vi "GM_MyRIO(FPGA).vi"() -> ()   [LabVIEW 2017]
uses:
  <vilib>/rvi/Emulation/niFpgaGetClockAttributes.vi
  <vilib>/rvi/Emulation/niFpgaSctlEmulationGetInTimedLoop.vi
  <vilib>/rvi/Emulation/niFpgaEmulationReportErrorSimple.vi
  <vilib>/rvi/interface/RandomDataEmulation/niFpgaRandomDataHandleErrors.vi
  <vilib>/rvi/Memory/Memory_Emulation/nirvimemoryEmulation.vi
  <vilib>/rvi/Memory/Memory_Emulation/nirvimemoryFastEmulation.vi
  <vilib>/rvi/DataTransferAndStorage/Container/Common/niFpgaContainerGetUniqueNameForEmu.vi
  <vilib>/rvi/Memory/Memory_Emulation/niFpgaMemoryEmulationCacheClearOnFirstRun.vi
  <vilib>/rvi/Memory/Memory_Emulation/nirvimemoryEmulationManagerCache_MakeExclusive.vi
  <vilib>/rvi/Memory/Memory_Emulation/niFpgaMemoryEmulationValidateCache.vi
  <vilib>/rvi/Memory/Memory_Emulation/nirvimemoryEmulationManagerCache_InsertValue.vi
  <vilib>/Utility/error.llb/Clear Errors.vi
  <vilib>/rvi/Memory/Memory_Emulation/nirvimemoryEmulationManagerCache_ReleaseExclusive.vi
  <vilib>/rvi/Memory/Memory_Emulation/nirvimemoryEmulationManagerCache_GetValue.vi
  <vilib>/rvi/Emulation/niFpgaEmulationIsFPGAContextNoSignature.vi
  <vilib>/rvi/Memory/Memory_Emulation/nirvimemoryEmulationManagerCache_SetValue.vi
  <vilib>/rvi/Emulation/niFpgaSctlEmulationResourceMgr.vi
  <vilib>/rvi/Emulation/niFpgaProcessEmulError.vi
  <vilib>/rvi/Emulation/niFpgaCriticalErrorInLSC.vi
  <vilib>/rvi/eio/common/nirviEmuTemplateMethod_errors.vi
  <vilib>/rvi/DataTransferAndStorage/Container/XNode/niFpgaContainer.xnode
  <vilib>/rvi/interface/RandomDataEmulation/nirviRandomDataFpgaReadWriteTemplate.vi
  <vilib>/eio/EIONode/EIONode.xnode
panel:
  in  "Zdiv":i8
  out "Zpre":u16
  out "Zbackpulse":i16
  in  "Zmotorbackspeedticks":u32
  out "XOUTCOUTN":u32
  out "Zoutnumber":u32
  in  "Zdir":bool
  in  "Xn-dz":u32
  in  "Zcount":u32
  in  "Stepm_pt_nm":u32
  in  "Laser/xn/dx":u32
  out "X out count":u32
  in  "FIFO_Timeout":i16
  in  "LaserNum":u32
  in  "delays":u32[](array[numeric])=[0, 0, 0, 0, 0, 0, 0, 0, 0, 0, 0, 0, 0, 0, 0, 0, 0, 0, 0, 0, 0, 0, 0, 0, 0, 0, 0, 0, 0, 0, 0, 0, 0, 0, 0, 0, 0, 0, 0, 0]
  in  "LsrCtrl":i32
  in  "VC_pt_nm":i16
  in  "LON":bool
  in  "Laserupdateus":u32 caption="Laserupdateus)"
  in  "stop 2":bool
  in  "VC_pt_in_fifo":i32
  in  "start_scan":bool
  in  "Ele_Ini_Dir":bool
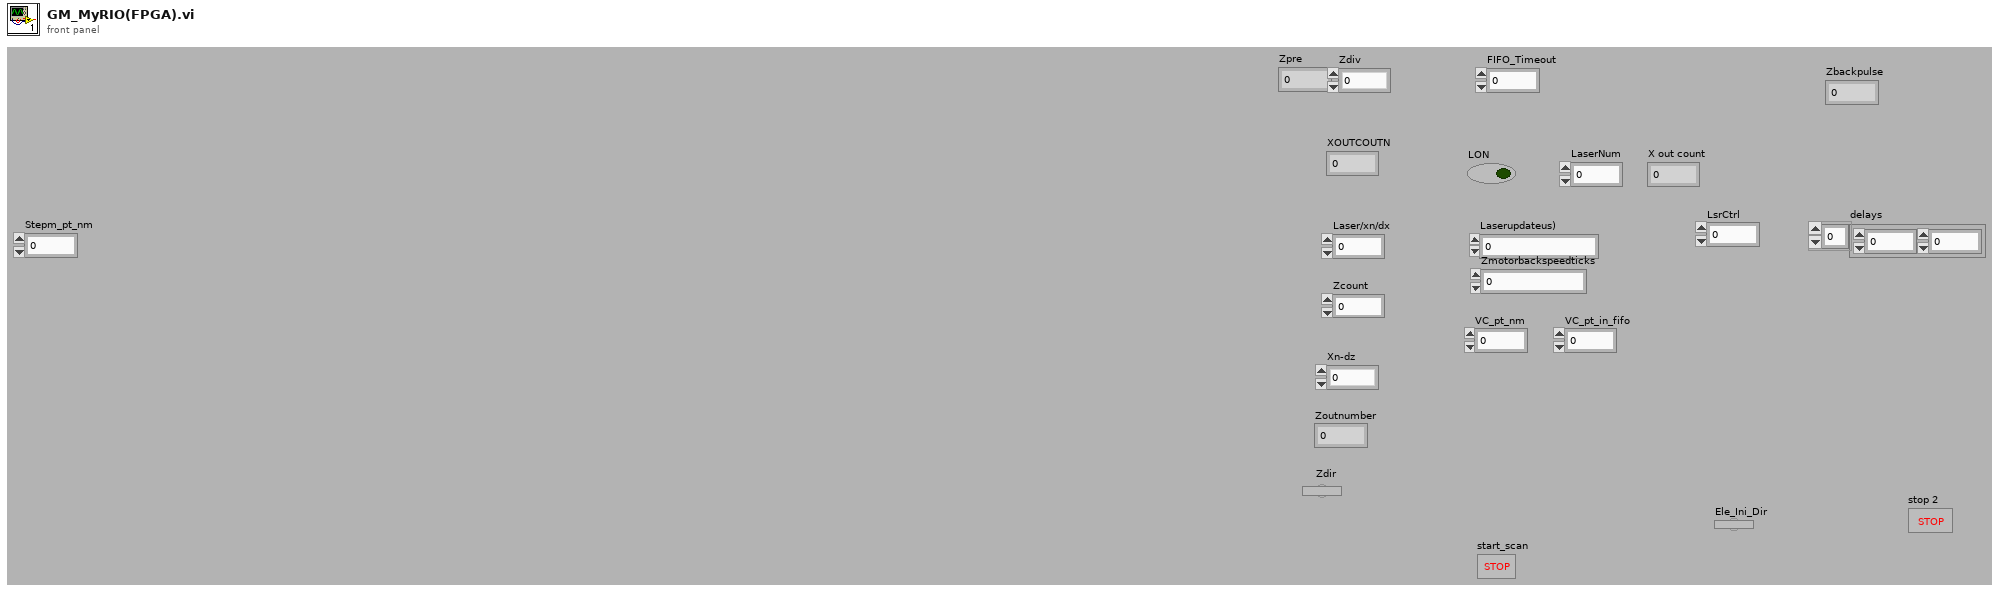
[diagram p1: front panel]
types:
  T1 = cluster{"Boolean array[0]":bool, "Boolean array[1]":bool, "Boolean array[2]":bool, "Boolean array[3]":bool, "Boolean array[4]":bool, "Boolean array[5]":bool, "Boolean array[6]":bool, "Boolean array[7]":bool, "Boolean array[8]":bool}
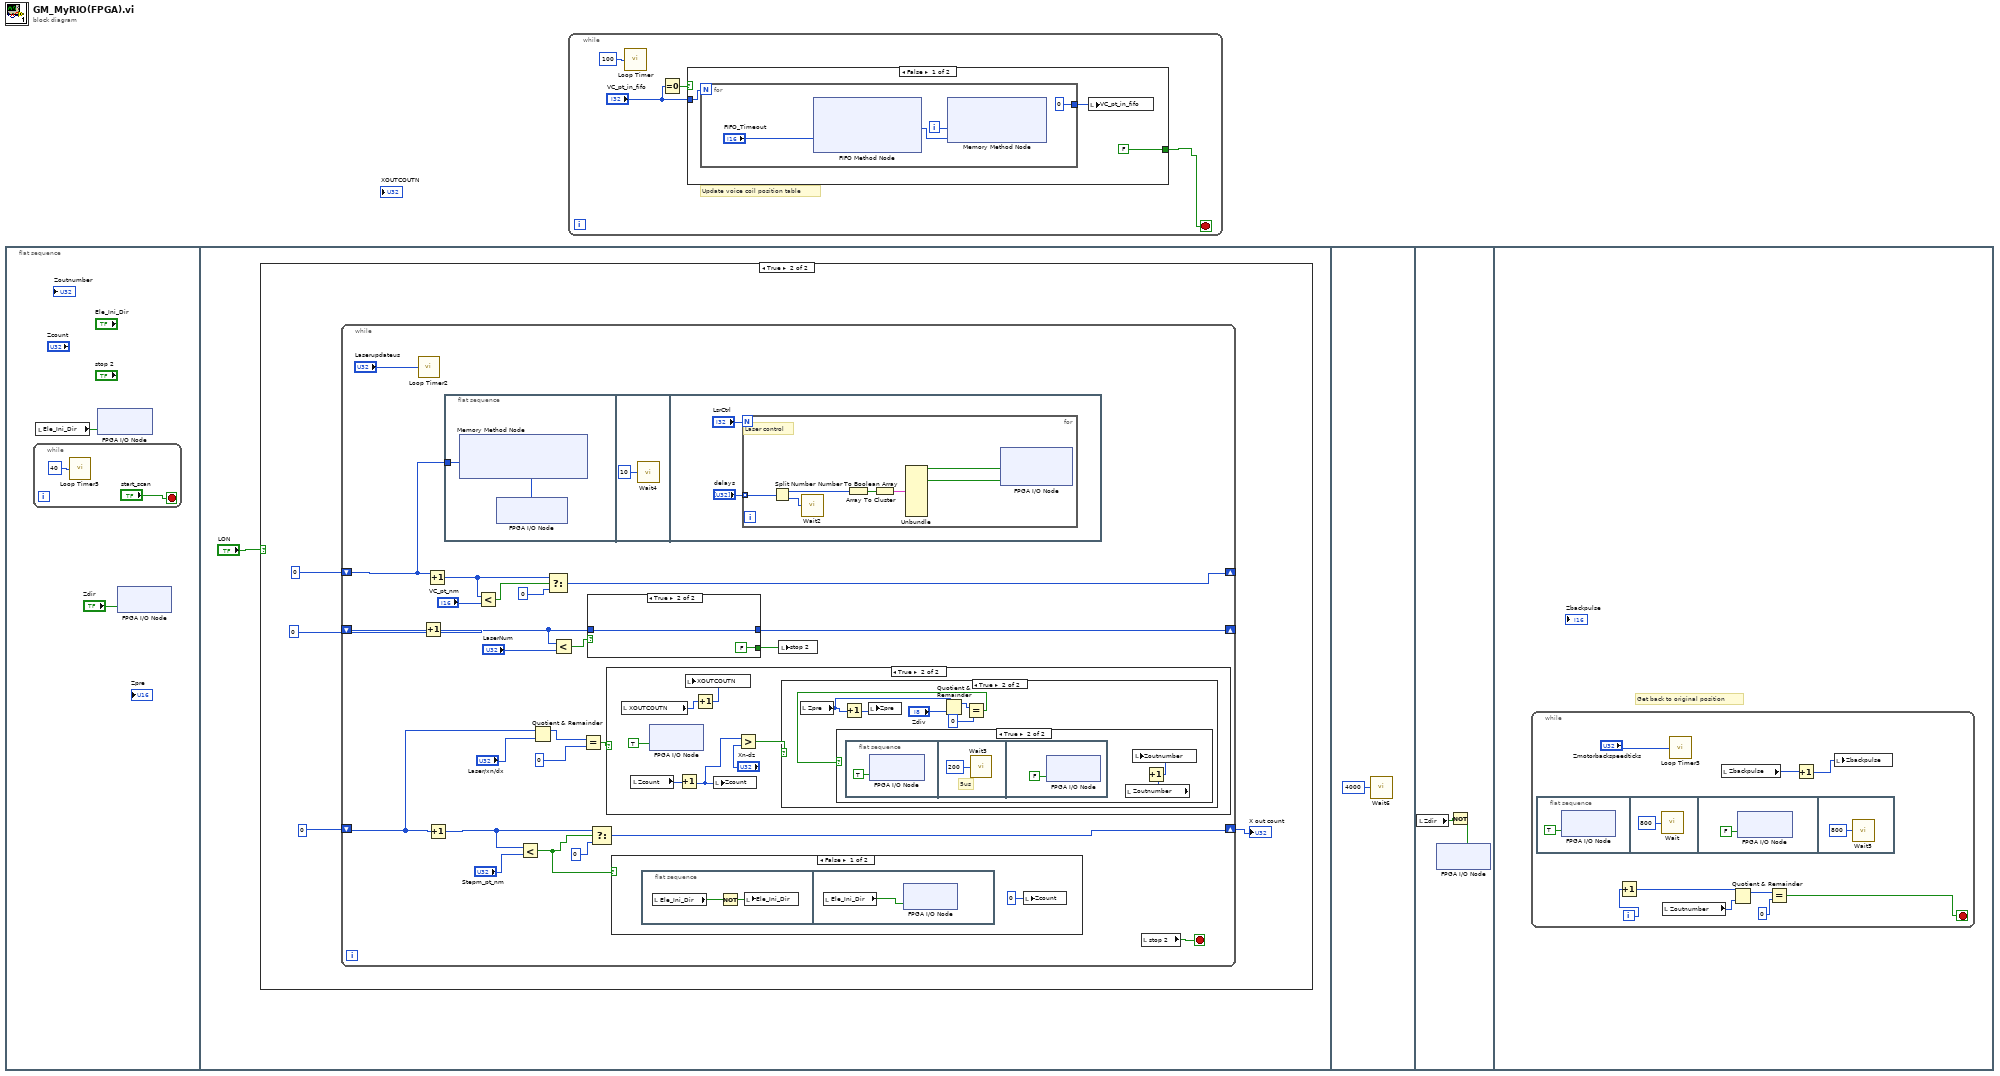
[diagram p0: block diagram]
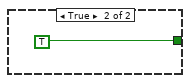
[diagram p2: hidden frame]
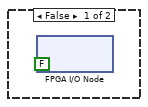
[diagram p4: hidden frame]
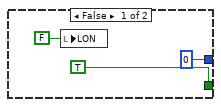
[diagram p8: hidden frame]
diagram:
  n1 = flat-sequence {
    frame #0 {
      n2 = while {
        stop <- "start_scan" stop-if-true
        n3 = call "Loop Timer5"("Count(Ticks)"=u8 40) -> ()  [unwired: 1 out]
      }
      n4 = local read "Ele_Ini_Dir"() -> (w2:bool)
      n5 = xnode "FPGA I/O Node"("X Dir"=w2) -> ()  [unwired: 1 in, 1 out]
      n6 = xnode "FPGA I/O Node"("Z Dir"="Zdir") -> ()  [unwired: 1 in, 1 out]
    }
    frame #1 {
      n7 = case shown="True" "LON" {
        frame False {
        }
        frame True {
          n8 = while {
            shift-right: [w31] -> _
            shift-left: 0 -> [w32]
            shift-right: [w29] -> _
            shift-left: 0 ("f") -> [w30]
            shift-right: [w16] -> w6
            shift-left: 0 -> [w10]
            stop <- w27 stop-if-true
            n9 = call "Loop Timer2"("Count(Ticks)"="Laserupdateus") -> ()  [unwired: 1 out]
            n10 = Increment(x=w32) -> (x+1=w24:i32)
            n11 = Increment(x=w30) -> (x+1=w20:i32)
            n12 = Increment(x=w10) -> (x+1=w15:i32)
            n13 = flat-sequence {
              tunnel: w30 -> [w57]
              frame #0 {
                n14 = xnode ("Memory Method Node")("Address"=w57) -> ("Data"=w58:i16)  [unwired: 1 in, 1 out]
                n15 = xnode "FPGA I/O Node"("Fast Mirror"=w58) -> ()  [unwired: 1 in, 1 out]
              }
              frame #1 {
                n16 = call "Wait4"("Count(Ticks)"=u8 10) -> ()  [unwired: 1 out]
              }
              frame #2 {
                n17 = for {
                  N: "LsrCtrl" -> [_]
                  tunnel: "delays" -> [w68] mode=indexing
                  # "Laser control"
                  n18 = Split Number(x=w68) -> (hi(x)=w65:u16, lo(x)=w64:u16)
                  n19 = call "Wait2"("Count(Ticks)"=w64) -> ()  [unwired: 1 out]
                  n20 = Number To Boolean Array(number=w65) -> (Boolean array=w67:bool[])
                  n21 = Array To Cluster(array=w67) -> (cluster=w66:T1)
                  n22 = Unbundle(w66) -> ("Boolean array[0]"=w63:bool, "Boolean array[2]"=w62:bool)  [unwired: 7 out]
                  n23 = xnode "FPGA I/O Node"("Laser1"=w63, "Daq trigger"=w62) -> ()  [unwired: 2 in, 2 out]
                }
              }
            }
            n24 = Less?(x=w20, y="VC_pt_nm") -> (x < y?=w23:bool)
            n25 = Less?(x=w15, y="Stepm_pt_nm") -> (x < y?=w17:bool)
            n26 = Quotient & Remainder(x=w10, y="Laser/xn/dx") -> (x-y*floor(x/y)=w13:u32)  [unwired: 1 out]
            n27 = Select(t=w20, s=w23, f=0) -> (s? t:f=w29:i32)
            n28 = Less?(x=w24, y="LaserNum") -> (x < y?=w25:bool)
            n29 = Equal?(x=w13, y=0) -> (x = y?=w11:bool)
            n30 = case shown="True" w25 {
              tunnel: w24 -> [_ w73]
              tunnel: [0 w73] -> w31
              tunnel: [TRUE FALSE] -> w28
              frame False {
                n31 = local write "LON"(FALSE ("LON")) -> ()
              }
              frame True {
              }
            }
            n32 = Select(t=w15, s=w17, f=0) -> (s? t:f=w16:i32)
            n33 = case shown="True" w11 {
              frame False {
                n34 = xnode "FPGA I/O Node"("X Step"=FALSE) -> ()  [unwired: 1 in, 1 out]
              }
              frame True {
                n35 = local read "XOUTCOUTN"() -> (w36:u32)
                n36 = local read "Zcount"() -> (w40:u32)
                n37 = xnode "FPGA I/O Node"("X Step"=TRUE) -> ()  [unwired: 1 in, 1 out]
                n38 = Increment(x=w40) -> (x+1=w39:u32)
                n39 = Increment(x=w36) -> (x+1=w35:u32)
                n40 = local write "XOUTCOUTN"(w35) -> ()
                n41 = local write "Zcount"(w39) -> ()
                n42 = Greater?(x=w39, y="Xn-dz") -> (0:w37:bool)
                n43 = case shown="True" w37 {
                  frame False {
                  }
                  frame True {
                    n44 = local read "Zpre"() -> (w46:u16)
                    n45 = Increment(x=w46) -> (x+1=w47:u16)
                    n46 = local write "Zpre"(w47) -> ()
                    n47 = Quotient & Remainder(x=w46, y="Zdiv") -> (x-y*floor(x/y)=w44:u16)  [unwired: 1 out]
                    n48 = Equal?(x=w44, y=i16 0) -> (x = y?=w42:bool)
                    n49 = case shown="True" w42 {
                      frame False {
                      }
                      frame True {
                        n50 = flat-sequence {
                          frame #0 {
                            n51 = xnode "FPGA I/O Node"("Z Step"=TRUE) -> ()  [unwired: 1 in, 1 out]
                          }
                          frame #1 {
                            # "5us"
                            n52 = call "Wait3"("Count(Ticks)"=u8 200) -> ()  [unwired: 1 out]
                          }
                          frame #2 {
                            n53 = xnode "FPGA I/O Node"("Z Step"=FALSE) -> ()  [unwired: 1 in, 1 out]
                          }
                        }
                        n54 = local read "Zoutnumber"() -> (w49:u32)
                        n55 = Increment(x=w49) -> (x+1=w48:u32)
                        n56 = local write "Zoutnumber"(w48) -> ()
                      }
                    }
                  }
                }
              }
            }
            n57 = case shown="False" w17 {
              frame False {
                n58 = flat-sequence {
                  frame #0 {
                    n59 = local read "Ele_Ini_Dir"() -> (w55:bool)
                    n60 = Not(x=w55) -> (.not. x?=w54:bool)
                    n61 = local write "Ele_Ini_Dir"(w54) -> ()
                  }
                  frame #1 {
                    n62 = local read "Ele_Ini_Dir"() -> (w56:bool)
                    n63 = xnode "FPGA I/O Node"("X Dir"=w56) -> ()  [unwired: 1 in, 1 out]
                  }
                }
                n64 = local write "Zcount"(u16 0 ("Zcount")) -> ()
              }
              frame True {
              }
            }
            n65 = local write "stop 2"(w28) -> ()
            n66 = local read "stop 2"() -> (w27:bool)
          }
          "X out count" <- w6
        }
      }
    }
    frame #2 {
      n67 = call "Wait6"("Count(Ticks)"=u16 4000) -> ()  [unwired: 1 out]
    }
    frame #3 {
      n68 = local read "Zdir"() -> (w76:bool)
      n69 = Not(x=w76) -> (.not. x?=w75:bool)
      n70 = xnode "FPGA I/O Node"("Z Dir"=w75) -> ()  [unwired: 1 in, 1 out]
    }
    frame #4 {
      # "Get back to original position"
      n71 = while {
        i -> [w84]
        stop <- w79 stop-if-true
        n72 = flat-sequence {
          frame #0 {
            n73 = xnode "FPGA I/O Node"("Z Step"=TRUE) -> ()  [unwired: 1 in, 1 out]
          }
          frame #1 {
            n74 = call "Wait"("Count(Ticks)"=u16 800) -> ()  [unwired: 1 out]
          }
          frame #2 {
            n75 = xnode "FPGA I/O Node"("Z Step"=FALSE) -> ()  [unwired: 1 in, 1 out]
          }
          frame #3 {
            n76 = call "Wait5"("Count(Ticks)"=u16 800) -> ()  [unwired: 1 out]
          }
        }
        n77 = Increment(x=w84) -> (x+1=w83:i32)
        n78 = local read "Zoutnumber"() -> (w82:u32)
        n79 = call "Loop Timer3"("Count(Ticks)"="Zmotorbackspeedticks") -> ()  [unwired: 1 out]
        n80 = local read "Zbackpulse"() -> (w78:i16)
        n81 = Quotient & Remainder(x=w83, y=w82) -> (x-y*floor(x/y)=w81:u32)  [unwired: 1 out]
        n82 = Equal?(x=w81, y=0) -> (x = y?=w79:bool)
        n83 = Increment(x=w78) -> (x+1=w77:i16)
        n84 = local write "Zbackpulse"(w77) -> ()
      }
    }
  }
  n85 = while {
    stop <- w90 stop-if-true
    # "Update voice coil position table"
    n86 = call "Loop Timer"("Count(Ticks)"=u8 100) -> ()  [unwired: 1 out]
    n87 = Equal To 0?(x="VC_pt_in_fifo") -> (x = 0?=w93:bool)
    n88 = case shown="False" w93 {
      tunnel: "VC_pt_in_fifo" -> [w96 _]
      tunnel: [FALSE TRUE] -> w90
      frame False {
        n89 = for {
          N: w96 -> [_]
          tunnel: [i16 0] -> w95
          i -> [w99]
          n90 = xnode ("FIFO Method Node")("Timeout"="FIFO_Timeout") -> ("Element"=w100:i16)  [unwired: 1 in, 2 out]
          n91 = xnode ("Memory Method Node")("Address"=w99, "Data"=w100) -> ()  [unwired: 1 in, 1 out]
        }
        n92 = local write "VC_pt_in_fifo"(w95) -> ()
      }
      frame True {
      }
    }
  }
